vi "trash_Version to String.vi"() -> ()   [LabVIEW 2021]
uses:
  Typedef/Version.ctl
  CIFCoreCommon.lvlib
panel:
  in  "Version":T1
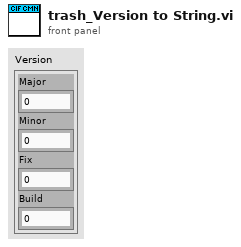
[diagram p1: front panel]
types:
  T1 = typedef "CIFCoreCommon.lvlib/Version.ctl" = cluster{"Major":i32, "Minor":i32, "Fix":i32, "Build":i32}
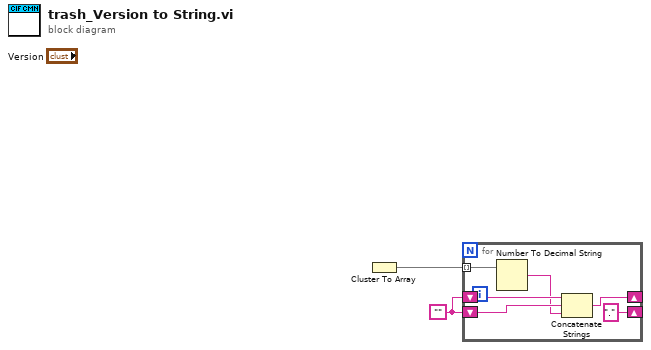
[diagram p0: block diagram]
diagram:
  w1 = ""
  n1 = Cluster To Array() -> (array=w2:void[])  [unwired: 1 in]
  n2 = for {
    tunnel: w2 -> [w6] mode=indexing
    shift-right: ["."] -> _
    shift-left: w1 -> [w7]
    shift-right: [w4] -> _
    shift-left: w1 -> [w8]
    n3 = Number To Decimal String(number=w6) -> (decimal integer string=w5:string)  [unwired: 1 in]
    n4 = Concatenate Strings(w8, w7, w5) -> (w4:string)
  }
